vi "Autolab Complete Example (B).vi"() -> ()   [LabVIEW 2011]
uses:
  C:/Program Files/Metrohm Autolab/Autolab SDK 1.10/EcoChemie.Autolab.Sdk.dll
  EcoChemie.Autolab.Sdk.dll
panel:
  out "PotentialApplied":dbl
  in  "Abort":bool
  in  "fileName":string
  out "IsMeasuring":bool
  in  "Save":bool
  in  "start measure":bool
  in  "Stop":bool
  out "XY Graph":cluster{"Y":dbl[], "Y":dbl[]}[](graph)
  out "X: WE(1).Potential":dbl
  out "Y: WE(1).Current":dbl
  out "P1 Port C read":u8
  out "ADC channel 3":dbl
  out "IsConnected":bool
  out "Cell":bool
  out "ManualCellSwitch":bool
  out "PotentialOverload":bool
  out "CurrentOverload":bool
  out "error out":errorcluster
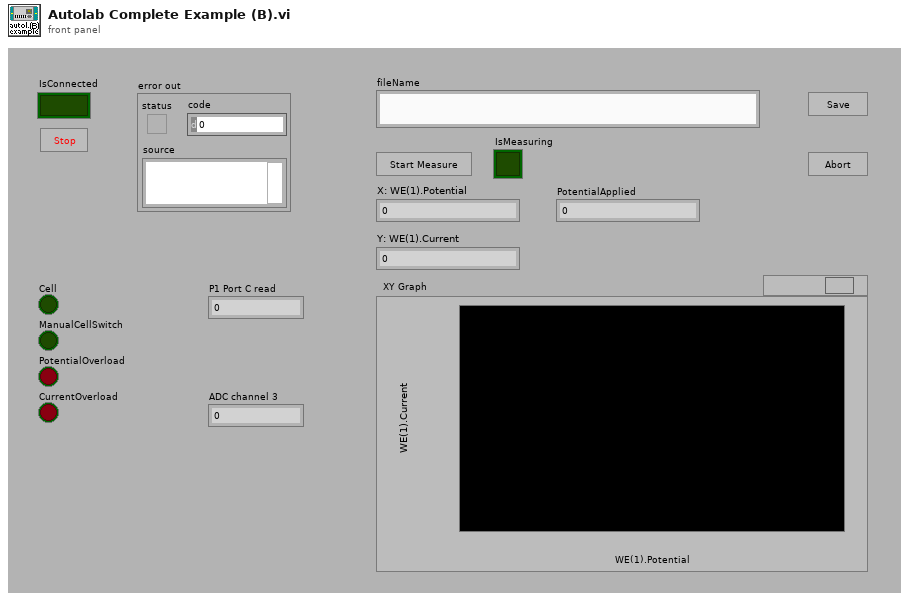
[diagram p1: front panel]
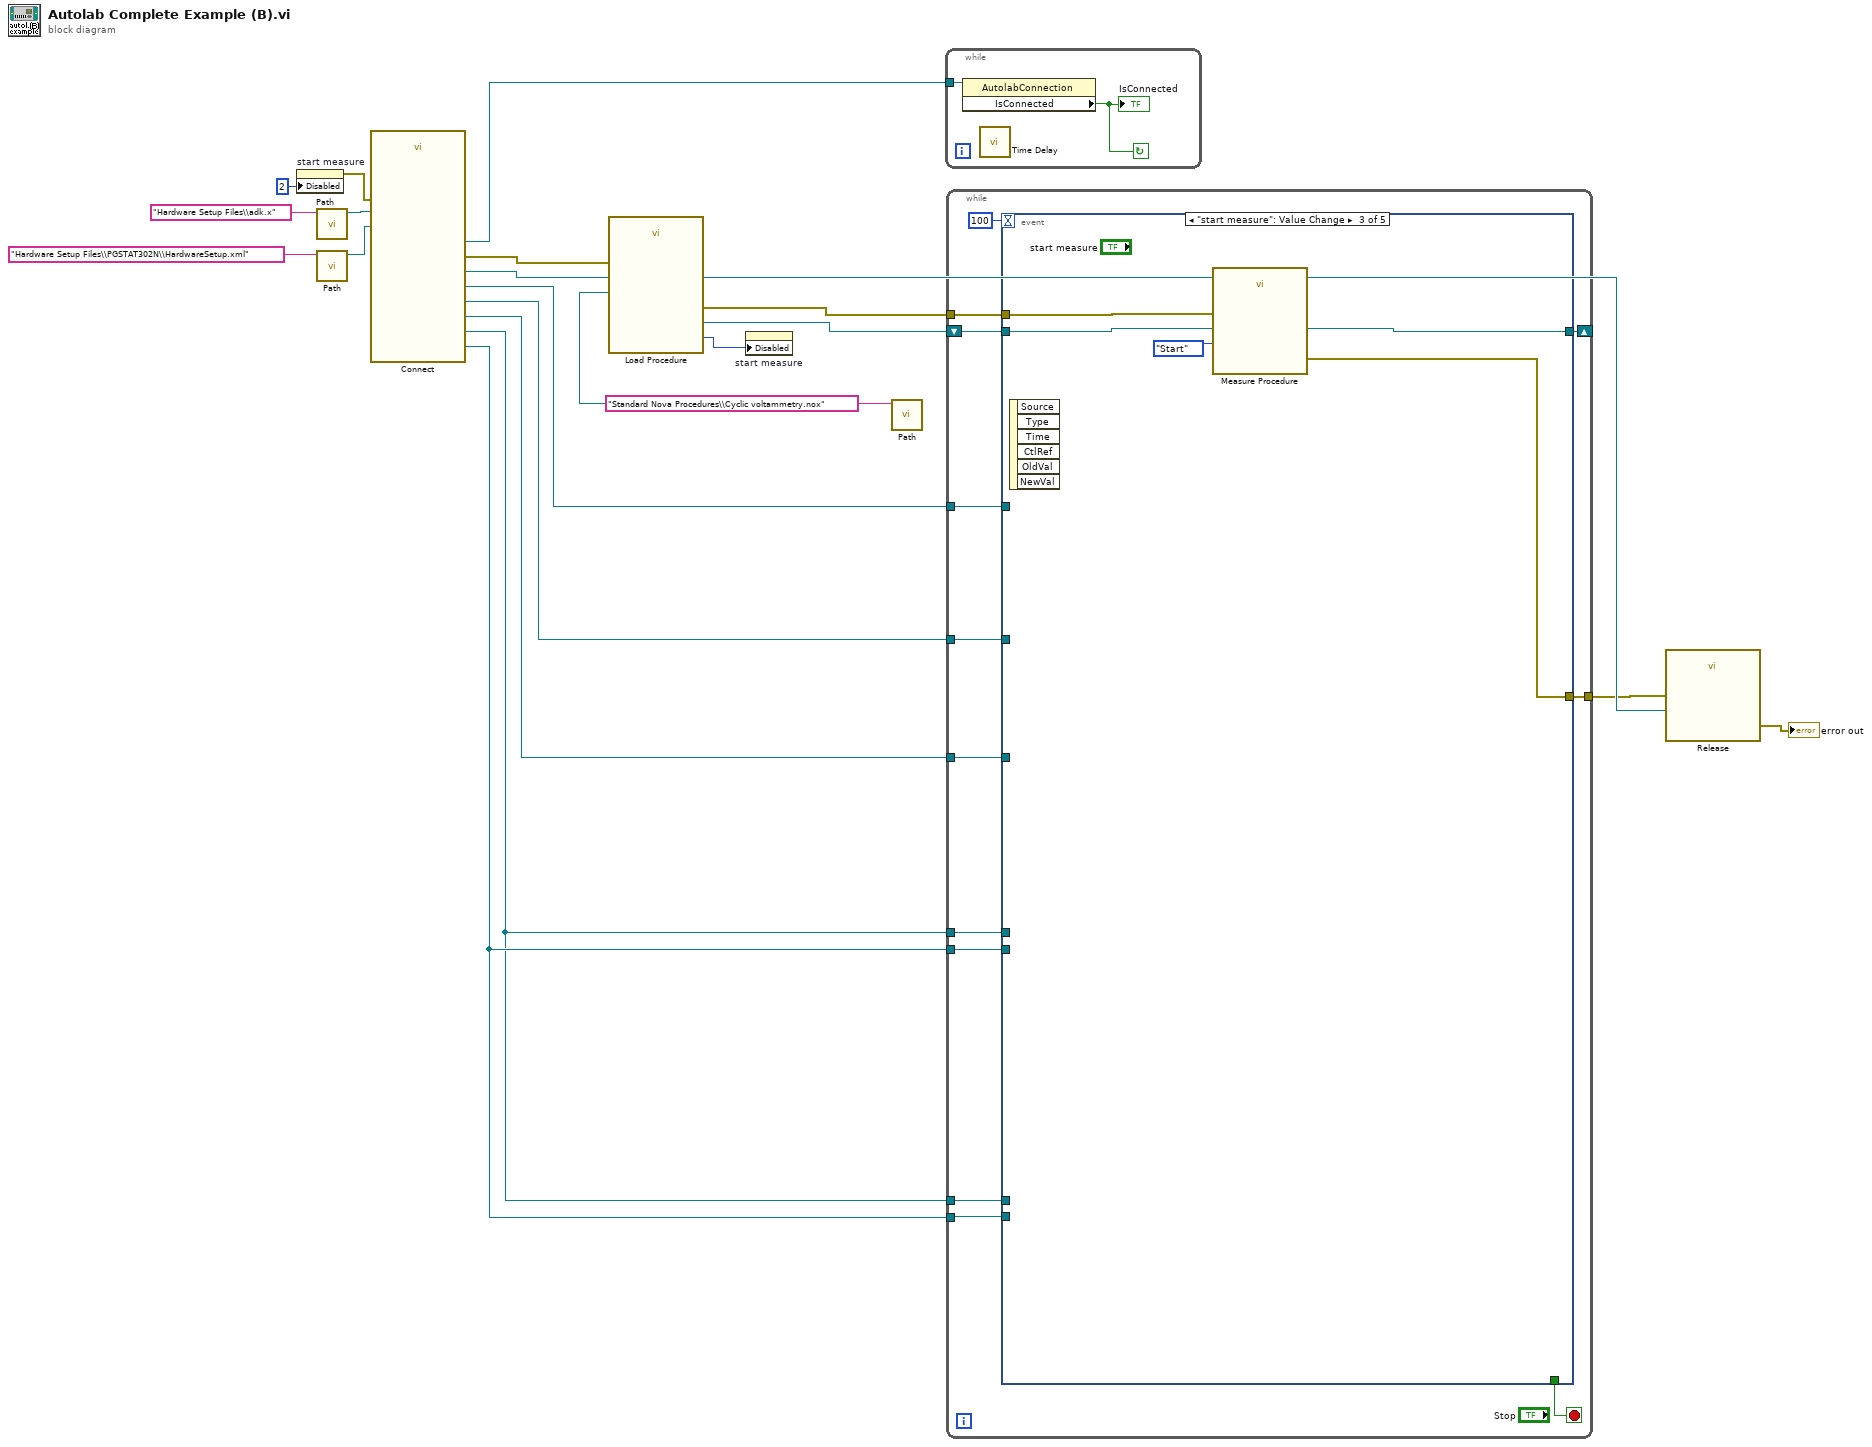
[diagram p0: block diagram]
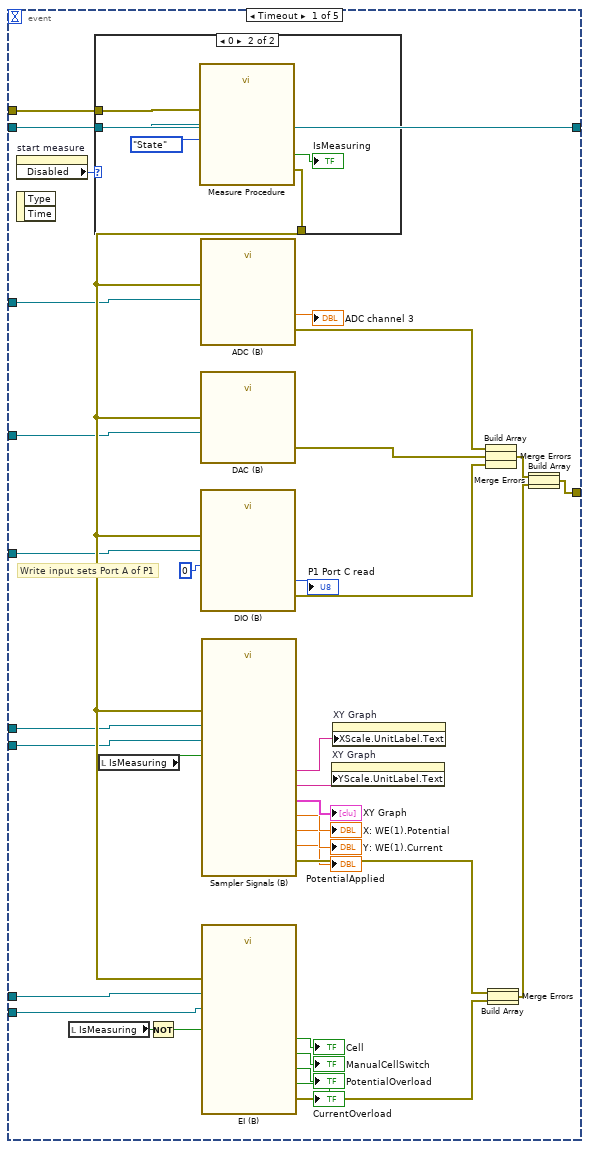
[diagram p2: hidden frame]
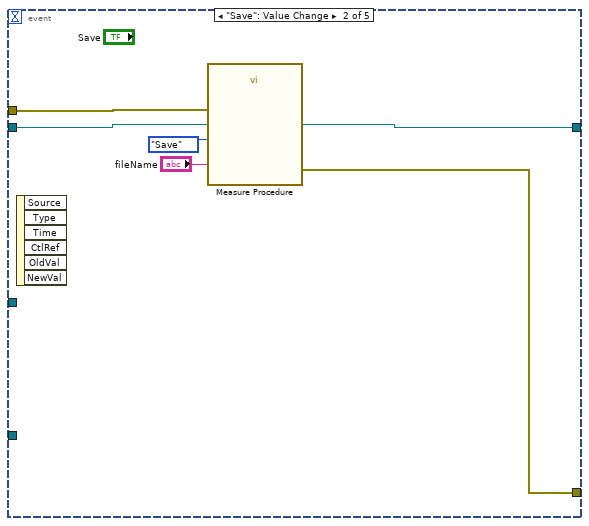
[diagram p4: hidden frame]
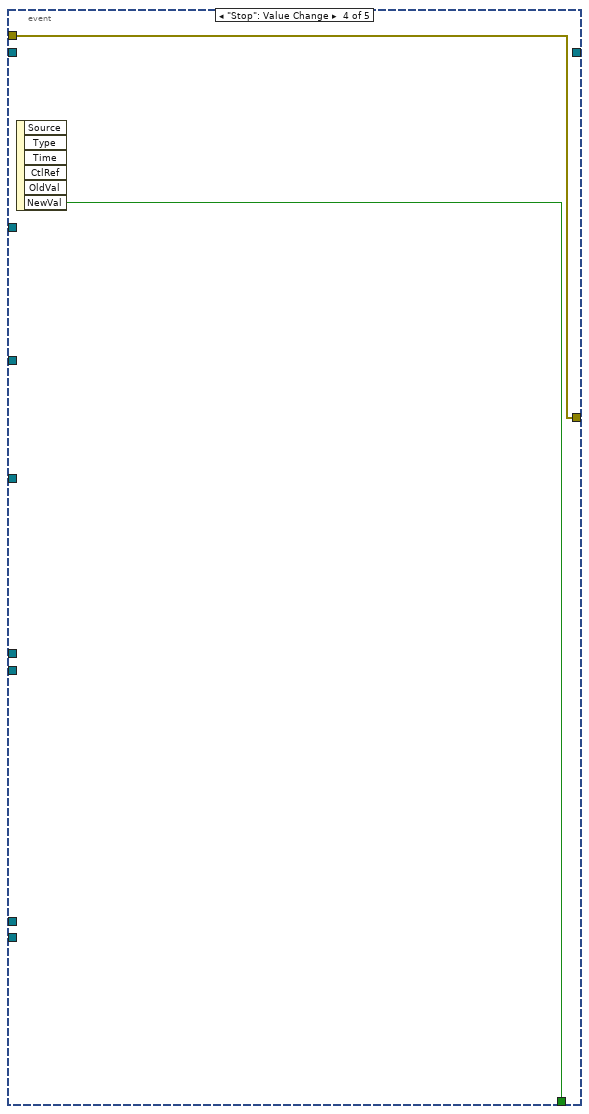
[diagram p5: hidden frame]
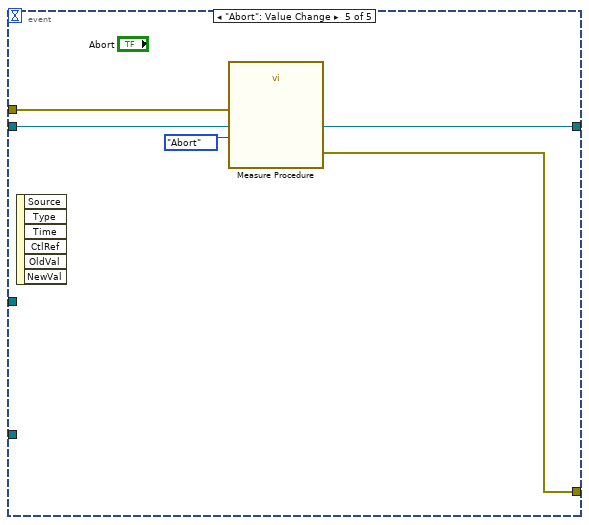
[diagram p6: hidden frame]
diagram:
  n1 = property on="start measure" class="Bool"("Disabled"=u8 2) -> (error out=w2:errorcluster)  [unwired: 2 in, 1 out]
  n2 = call "Path.vi"("name or relative path"="Hardware Setup Files\\adk.x") -> ("appended path"=w17:path)  [unwired: 10 in]
  n3 = call "Path.vi"("name or relative path"="Hardware Setup Files\\PGSTAT302N\\HardwareSetup.xml") -> ("appended path"=w16:path)  [unwired: 10 in]
  n4 = call "Connect.vi"("Embedded Exe File"=w17, "Hardware Setup File"=w16, "error in (no error)"=w2) -> ("Adc"=w8:refnum<k24>, "Dac"=w7:refnum<k24>, "Dio"=w6:refnum<k24>, "Sampler"=w4:refnum<k24>, "AutolabConnection"=w21:refnum<k24>, "instrument"=w12:refnum<k24>, "Ei"=w5:refnum<k24>, "error out"=w14:errorcluster)  [unwired: 5 in]
  n5 = call "Path.vi"("name or relative path"="Standard Nova Procedures\\Cyclic voltammetry.nox") -> ("appended path"=w13:path)  [unwired: 10 in]
  n6 = call "Load Procedure.vi"("error in (no error)"=w14, "Procedure"=w13, "Instrument"=w12) -> ("error out"=w3:errorcluster, "Numeric"=w11:i32, "LoadProcedure"=w10:refnum<k24>)  [unwired: 5 in, 1 out]
  n7 = property on="start measure" class="Bool"("Disabled"=w11) -> ()  [unwired: 2 in, 2 out]
  n8 = while {
    tunnel: w21 -> [w22]
    stop <- w23 continue-if-true
    n9 = property class="AutolabConnection"(reference=w22) -> ("IsConnected"=w23:bool)  [unwired: 1 in, 2 out]
    "IsConnected" <- w23
    n10 = call "Time Delay"() -> ()  [unwired: 11 in, 1 out]
  }
  n11 = while {
    shift-right: [w36] -> _
    shift-left: w10 -> [w35]
    tunnel: [w34] -> w9
    tunnel: w8 -> [w33]
    tunnel: w7 -> [w32]
    tunnel: w6 -> [w31]
    tunnel: w4 -> [w30]
    tunnel: w5 -> [w29]
    tunnel: w4 -> [w28]
    tunnel: w5 -> [w27]
    tunnel: w3 -> [w26]
    stop <- w25 stop-if-true
    n12 = event shown="[2] \"start measure\": Value Change" {
      selector: _ -> [_ _ _ _ _]
      dyn-events: _ -> [_ _ _ _ _]
      timeout: 100 -> [_ _ _ _ _]
      tunnel: [w40 w81 w89 _ w94] -> w36
      tunnel: w35 -> [w40 w81 w89 _ w94]
      tunnel: [w49 w82 w88 w90 w93] -> w34
      tunnel: w33 -> [w48 _ _ _ _]
      tunnel: w32 -> [w47 _ _ _ _]
      tunnel: w31 -> [w46 _ _ _ _]
      tunnel: w30 -> [w45 _ _ _ _]
      tunnel: w29 -> [w44 _ _ _ _]
      tunnel: w28 -> [w43 _ _ _ _]
      tunnel: w27 -> [w42 _ _ _ _]
      tunnel: w26 -> [w41 w83 w87 w90 w95]
      tunnel: [_ _ _ w91 _] -> w25
      event Timeout {
        # "Write input sets Port A of P1"
        n13 = property on="start measure" class="Bool"() -> ("Disabled"=w51:u8)  [unwired: 2 in, 2 out]
        n14 = event-data() -> ()  [unwired: 1 in, 2 out]
        n15 = local read "IsMeasuring"() -> (w73:bool)
        n16 = case shown="0" w51 {
          tunnel: w40 -> [_ w78]
          tunnel: [w75 w77] -> w50
          tunnel: w41 -> [w75 w76]
          frame 2, Default {
          }
          frame 0 {
            n17 = call "Measure Procedure.vi"("error in"=w76, "Request for procedure"=enum16{"State", "Save", "Abort", "Start"}."State", "LoadProcedure"=w78) -> ("error out"=w77:errorcluster, "IsMeasuring"=→"IsMeasuring":bool)  [unwired: 7 in]
          }
        }
        n18 = local read "IsMeasuring"() -> (w59:bool)
        n19 = Not(x=w73) -> (.not. x?=w69:bool)
        n20 = call "ADC (B).vi"("error in"=w50, "Adc"=w48) -> ("error out"=w56:errorcluster, "Sample"=→"ADC channel 3":dbl)  [unwired: 8 in]
        n21 = call "DAC (B).vi"("error in (no error)"=w50, "Dac"=w47) -> ("error out"=w55:errorcluster)  [unwired: 9 in]
        n22 = call "DIO (B).vi"("error in (no error)"=w50, "Write"=u8 0, "DIO"=w46) -> ("error out"=w54:errorcluster, "Read"=→"P1 Port C read":u8)  [unwired: 7 in]
        n23 = call "Sampler Signals (B).vi"("Sampler"=w45, "EI"=w44, "measure"=w59, "error in"=w50) -> ("X"=→"X: WE(1).Potential":dbl, "Y"=→"Y: WE(1).Current":dbl, "Signal X"=w60:string, "XY Graph"=→"XY Graph":cluster{"Y":dbl[], "Y":dbl[]}[], "Signal Y"=w61:string, "PotentialApplied"=→"PotentialApplied":dbl, "error out"=w74:errorcluster)  [unwired: 5 in]
        n24 = call "EI (B).vi"("Ei"=w42, "Sampler"=w43, "Disable Sampler"=w69, "error in (no error)"=w50) -> ("CurrentOverload"=→"CurrentOverload":bool, "PotentialOverload"=→"PotentialOverload":bool, "Cell"=→"Cell":bool, "ManualCellSwitch"=→"ManualCellSwitch":bool, "error out"=w57:errorcluster)  [unwired: 11 in]
        n25 = property on="XY Graph" class="XYGraph (strict)"("YScale.UnitLabel.Text"=w61) -> ()  [unwired: 2 in, 2 out]
        n26 = property on="XY Graph" class="XYGraph (strict)"("XScale.UnitLabel.Text"=w60) -> ()  [unwired: 2 in, 2 out]
        n27 = Build Array(w56, w55, w54) -> (w39:errorcluster[])
        n28 = Merge Errors(w39) -> (w53:errorcluster)
        n29 = Build Array(w74, w57) -> (w38:errorcluster[])
        n30 = Merge Errors(w38) -> (w52:errorcluster)
        n31 = Build Array(w53, w52) -> (w37:errorcluster[])
        n32 = Merge Errors(w37) -> (w49:errorcluster)
      }
      event "Save": Value Change {
        n33 = event-data() -> ()  [unwired: 1 in, 6 out]
        n34 = call "Measure Procedure.vi"("error in"=w83, "fileName"="fileName", "Request for procedure"=enum16{"State", "Save", "Abort", "Start"}."Save", "LoadProcedure"=w81) -> ("error out"=w82:errorcluster)  [unwired: 6 in, 1 out]
      }
      event "start measure": Value Change {
        n35 = event-data() -> ()  [unwired: 1 in, 6 out]
        n36 = call "Measure Procedure.vi"("error in"=w87, "Request for procedure"=enum16{"State", "Save", "Abort", "Start"}."Start", "LoadProcedure"=w89) -> ("error out"=w88:errorcluster)  [unwired: 7 in, 1 out]
      }
      event "Stop": Value Change {
        n37 = event-data() -> ("NewVal"=w91:bool)  [unwired: 1 in, 5 out]
      }
      event "Abort": Value Change {
        n38 = event-data() -> ()  [unwired: 1 in, 6 out]
        n39 = call "Measure Procedure.vi"("error in"=w95, "Request for procedure"=enum16{"State", "Save", "Abort", "Start"}."Abort", "LoadProcedure"=w94) -> ("error out"=w93:errorcluster)  [unwired: 7 in, 1 out]
      }
    }
  }
  n40 = call "Release.vi"("error in (no error)"=w9, "Instrument"=w12) -> ("error out"=→"error out":errorcluster)  [unwired: 9 in]
